vi "ToTable.vi"(8 "error in":errorcluster, 9 "Table Index":i32, 10 "variant":variant, 11 "OPC UA editor node in":refnum<class "OPC UA Client editor node.lvclass">) -> (0 "error out":errorcluster, 1 "headers":string[](array[string]), 2 "table":string[][](array[string]), 3 "OPC UA editor node out":refnum<class "OPC UA Client editor node.lvclass">)   [LabVIEW 2013, in "OPC UA Client editor node.lvclass"]
doc: "Copyright 2015 National Instruments Corporation\n\nLicensed under the Apache License, Version 2.0 (the \"License\"); you may not use this file except in compliance with the License. You may obtain a copy of the License at http://www.apache.org/licenses/LICENSE-2.0\nUnless required by applicable law or agreed to in writing, software distributed under the License is distributed on an \"AS IS\" BASIS, WITHOUT WARRANTIES OR CONDITIONS OF ANY KIND, either express or implied. See the License for the specific language governing permissions and limitations under the License."
uses:
  OPC UA Client editor node.lvclass
  module/configuration/OPC UA Client configuration.lvclass
  <vilib>/NI/Module Execution Interface/Engine Configuration/engine configuration.lvclass
  module/configuration/OPC UA Client configuration.lvclass/OPC UA Client configuration.ctl
  <vilib>/NI/Configuration Framework/serializable configuration/NISE_CEF_serializable configuration.lvclass/NISE_CEF_serializable configuration.ctl
  <vilib>/NI/Tag Bus/tag/tag descriptor.lvclass/tag descriptor.ctl
  <vilib>/NI/Tag Bus Module Framework/channel/TBM channel.lvclass/TBM channel.ctl
  module/configuration/Read Lines.vi
  <vilib>/Utility/LVClass/Get LV Class Name.vi
  <vilib>/NI/Configuration Framework/error generator/NISE_error generator.vi
  <vilib>/NI/Tag Bus/tag/tag descriptor.lvclass
  <vilib>/NI/Tag Bus Module Framework/channel/TBM channel.lvclass
  <vilib>/NI/Configuration Framework/serializable configuration/NISE_CEF_serializable configuration.lvclass
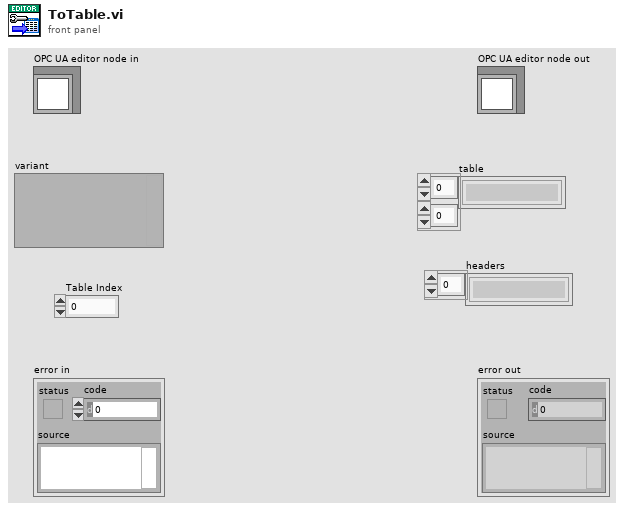
[diagram p1: front panel]
types:
  T1 = typedef "OPC UA configuration.lvclass/Line.ctl" = cluster{"channel":refnum<class "TBM channel.lvclass">, "Node Path":string, "OPC UA Data Type":T2}
  T2 = typedef "OPC UA configuration.lvclass/OPC UA Data Type.ctl" = u16
  T3 = typedef "OPC UA Client editor node.lvclass/OPC UA DataType Enum.ctl" = enum16{"Boolean", "SByte", "Byte", "Int16", "UInt16", "Int32", "UInt32", "Int64", "UInt64", "Float", "Double", "String", "DateTime", "ByteString", "Array of Boolean", "Array of SByte", "Array of Byte", "Array of Int16", "Array of UInt16", "Array of Int32", "Array of UInt32", "Array of Int64", "Array of UInt64", "Array of Float", "Array of Double", "Array of String", "Array of DateTime"}
  T4 = typedef "TBM channel.lvclass/channel classification.ctl" = enum16{"input data", "output data", "processing parameter", "processing result"}
  T5 = typedef "tag bus.lvlib/tag descriptor.lvclass/Data Type.ctl" = enum16{"Double", "Single", "I64", "I32", "I16", "I8", "U64", "U32", "U16", "U8", "Boolean", "String", "Array of Double", "Array of Single", "Array of I64", "Array of I32", "Array of I16", "Array of I8", "Array of U64", "Array of U32", "Array of U16", "Array of U8", "Array of Boolean", "Array of String"}
  T6 = typedef "OPC UA Client editor node.lvclass/permissions.ctl" = enum32{"Read from HW", "Write to HW"}
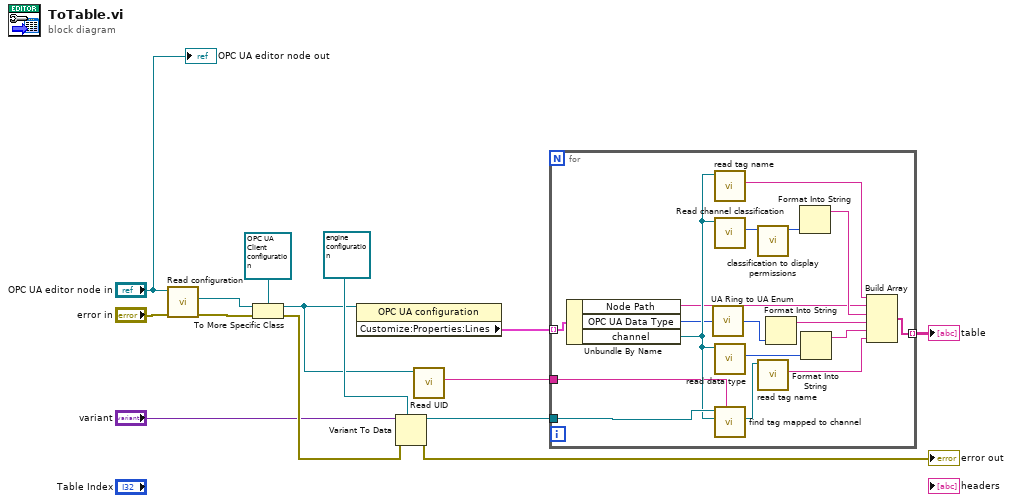
[diagram p0: block diagram]
diagram:
  n1 = call-dynamic "Read configuration.vi"("error in"="error in", "OPC UA editor node in"="OPC UA editor node in") -> ("error out"=w14:errorcluster, "configuration"=w6:refnum<class "NISE_CEF_serializable configuration.lvclass">)  [unwired: 7 in, 1 out]
  n2 = To More Specific Class(target class=refnum<class "OPC UA Client configuration.lvclass"> refnum ("tag bus configurable plugin module configuration"), reference=w6, error in=w14) -> (specific class reference=w5:refnum<class "OPC UA Client configuration.lvclass">, error out=w3:errorcluster)
  n3 = property class="OPC UA configuration"(reference=w5) -> ("Customize:Properties:Lines"=w11:T1[])  [unwired: 1 in, 2 out]
  n4 = Variant To Data(error in=w3, type=refnum<class "engine configuration.lvclass"> refnum ("engine configuration"), Variant="variant") -> (data=w9:refnum<class "engine configuration.lvclass">, error out=→"error out":errorcluster)
  n5 = call <vilib>:"Read UID.vi"("configuration in"=w5) -> ("instance id"=w4:string)  [unwired: 8 in, 2 out]
  n6 = for {
    tunnel: w11 -> [w31] mode=indexing
    tunnel: w9 -> [w30]
    tunnel: [w23] -> w7 mode=indexing
    tunnel: w4 -> [w22]
    n7 = Unbundle By Name(w31) -> ("Node Path"=w18:string, "OPC UA Data Type"=w15:T2, "channel"=w25:refnum<class "TBM channel.lvclass">)
    n8 = call "UA Ring to UA Enum.vi"("OPC UA Data Type Ring"=w15) -> ("OPC Data Type Enum"=w16:T3)
    n9 = call <vilib>:"read tag name.vi"("system tag in"=w25) -> ("name"=w21:string)  [unwired: 8 in, 2 out]
    n10 = call <vilib>:"Read channel classification.vi"("channel in"=w25) -> ("channel classification"=w28:T4)  [unwired: 8 in, 2 out]
    n11 = call <vilib>:"read data type.vi"("system tag in"=w25) -> ("data type"=w24:T5)  [unwired: 8 in, 2 out]
    n12 = call <vilib>:"find tag mapped to channel.vi"("owner"=w22, "channel"=w25, "engine configuration in"=w30) -> ("tag"=w29:refnum<class "tag descriptor.lvclass">)  [unwired: 6 in, 2 out]
    n13 = call "classification to display permissions.vi"("channel classification"=w28) -> ("permissions"=w27:T6)  [unwired: 10 in]
    n14 = call <vilib>:"read tag name.vi"("system tag in"=w29) -> ("name"=w20:string)  [unwired: 8 in, 2 out]
    n15 = Format Into String(w16) -> (resulting string=w17:string)  [unwired: 3 in, 1 out]
    n16 = Format Into String(w27) -> (resulting string=w26:string)  [unwired: 3 in, 1 out]
    n17 = Format Into String(w24) -> (resulting string=w19:string)  [unwired: 3 in, 1 out]
    n18 = Build Array(w21, w18, w26, w17, w19, w20) -> (w23:string[])
  }
  "table" <- w7
  "OPC UA editor node out" <- "OPC UA editor node in"
